vi "myRIO_BRig_RT_dataBlock_BTPR__L.vi"() -> (2 "output_BTPR__L":i32)   [LabVIEW 2014]
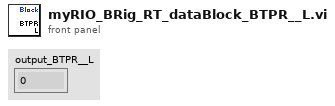
[diagram p1: front panel]
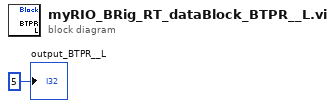
[diagram p0: block diagram]
diagram:
  "output_BTPR__L" <- 5 ("output_iBlock")
